vi "TDMS Channel Page.vi"(8 "error in (no error)":errorcluster, 11 "Node Ptr":T2 format="%.0x") -> (0 "error out":errorcluster)   [LabVIEW 2011, in "TDMS Custom Device.lvlib"]
uses:
  TDMS Custom Device.lvlib
  <vilib>/NI Veristand/Custom Device API/Custom Device Item Ref.ctl
  <vilib>/NI Veristand/Custom Device API/Get Item Property (Double).vi
  <vilib>/NI Veristand/Custom Device API/Get Item Property (I32).vi
  <vilib>/NI Veristand/Custom Device API/Get Item Property (Variant).vi
  <vilib>/NI Veristand/Custom Device API/Set Item Property (Double).vi
  <vilib>/NI Veristand/Custom Device API/Set Item Property (I32).vi
  <vilib>/NI Veristand/Custom Device API/Set Item Property (Variant).vi
  <vilib>/NI Veristand/Custom Device API/Custom Device API.lvlib
panel:
  in  "dt (sec)":dbl
  in  "Interpolation Width":i32=1 caption="The system uses this number of samples on either side of a point to be used by the above method. Increase to increase smoothness, decrease for performance." min=1 max=50
  in  "Interpolation Method":T1(ring)=enum."Linear"
  in  "Header":cluster{"Section Name":string}={"Section Name"="TDMS Channel Settings"}
  in  "Description":string
  out "Name":string
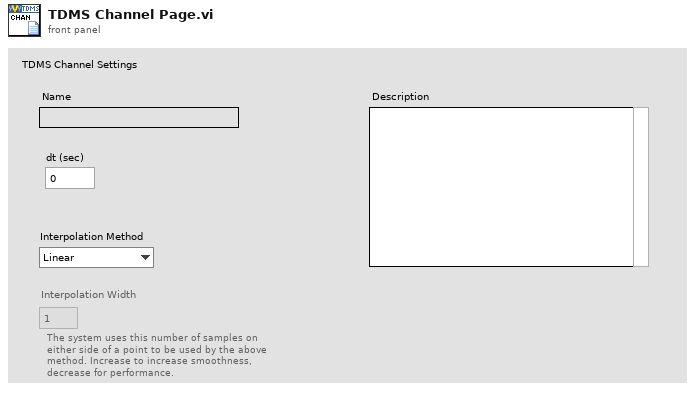
[diagram p1: front panel]
types:
  T1 = enum16{"Nearest", "Linear", "Spline", "Cubic Hermite", "Lagrange", "Polynomial"}
  T2 = typedef "Custom Device API.lvlib/Custom Device Item Ref.ctl" = u64
  T3 = enum8{"Enabled", "Disabled", "Disabled and Grayed Out"}
  T4 = typedef "Custom Device API.lvlib/Custom Device Item Info.ctl" = cluster{"Name":string, "Is Channel":bool, "GUID":string}
  T5 = typedef "Custom Device API.lvlib/Custom Device Commands.ctl" = enum16{"Default", "Item renamed", "Shutdown", "Dynamic button pressed"}
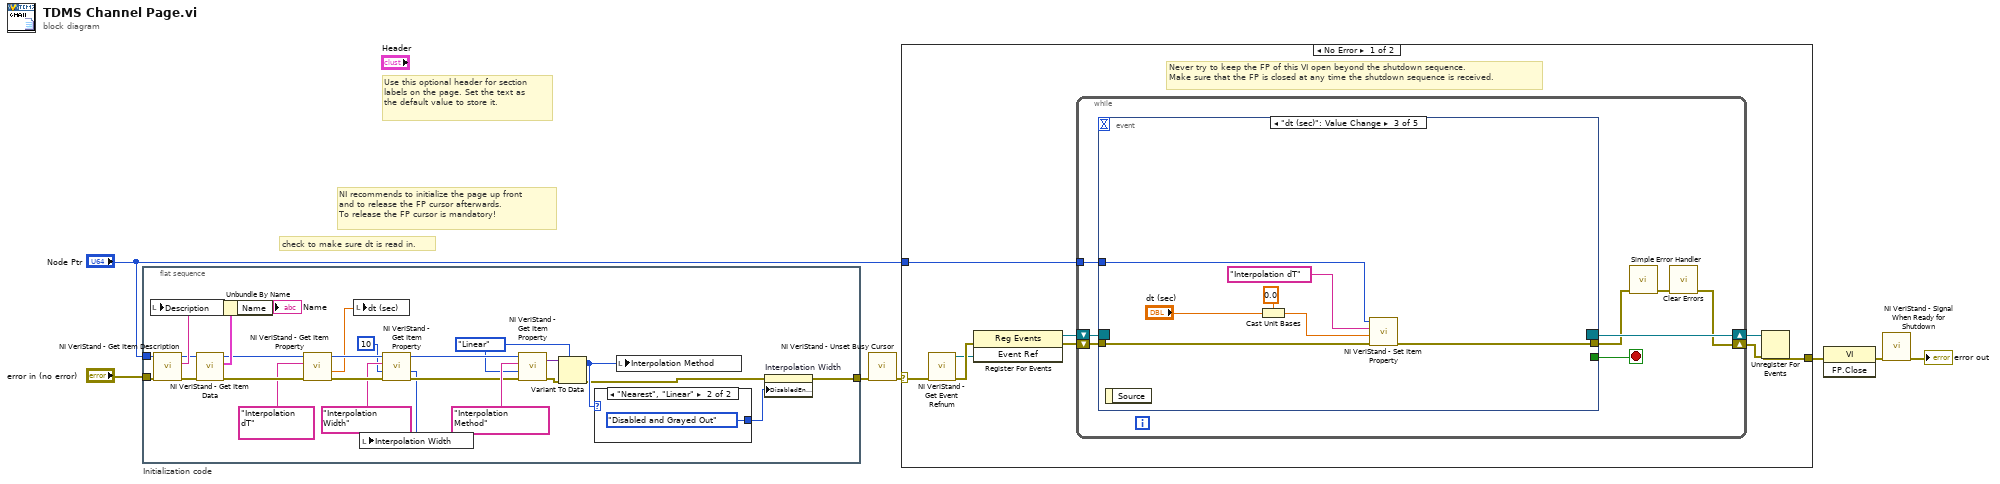
[diagram p0: block diagram]
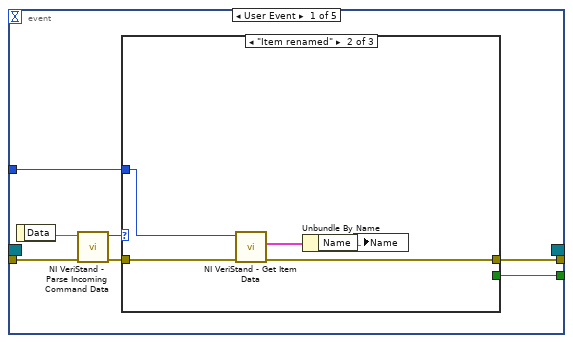
[diagram p2: hidden frame]
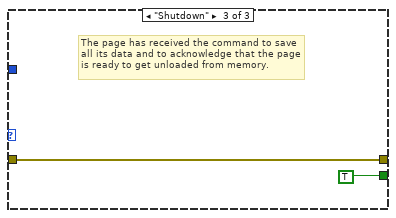
[diagram p4: hidden frame]
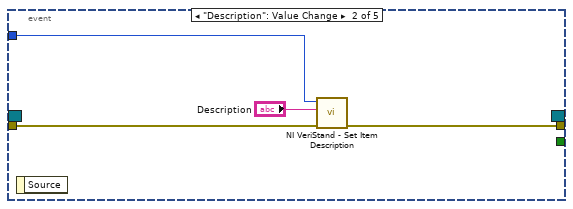
[diagram p5: hidden frame]
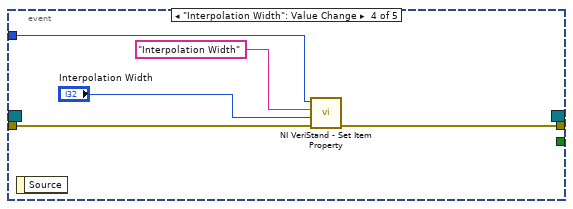
[diagram p6: hidden frame]
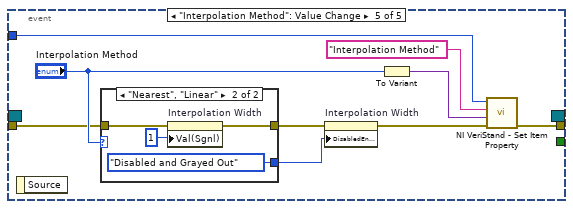
[diagram p7: hidden frame]
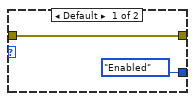
[diagram p8: hidden frame]
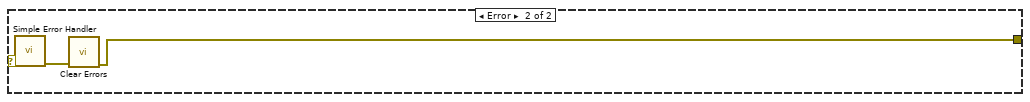
[diagram p9: hidden frame]
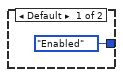
[diagram p10: hidden frame]
diagram:
  # "check to make sure dt is read in."
  # "Use this optional header for section labels on the page. Set the text as the default value to store it."
  # "NI recommends to initialize the page up front\nand to release the FP cursor afterwards.\nTo release the FP cursor is mandatory!"
  n1 = flat-sequence "Initialization code" {
    tunnel: "error in (no error)" -> [w33]
    tunnel: "Node Ptr" -> [w32]
    tunnel: [w12] -> w1
    frame #0 {
      w14 = T1."Linear" ("Interpolation Method")
      n2 = call <vilib>:"NI VeriStand - Get Item Description.vi"("error in (no error)"=w33, "Item Ref in"=w32) -> ("error out"=w30:errorcluster, "Description"=w31:string, "Item Ref out"=w29:T2)  [unwired: 7 out]
      n3 = local write "Description"(w31) -> ()
      n4 = call <vilib>:"NI VeriStand - Get Item Data.vi"("error in (no error)"=w30, "Item Ref in"=w29) -> ("error out"=w26:errorcluster, "Item Info"=w28:T4, "Item Ref out"=w27:T2)  [unwired: 7 out]
      n5 = Unbundle By Name(w28) -> ("Name"=→"Name":string)
      n6 = call-poly <vilib>:"NI VeriStand - Get Item Property.vi"("error in (no error)"=w26, "Property Name"="Interpolation dT", "Item Ref in"=w27) -> ("error out"=w20:errorcluster, "Value"=w8:dbl, "Item Ref out"=w19:T2)  [unwired: 1 in, 5 out]
      n7 = local write "dt (sec)"(w8) -> ()
      n8 = call-poly <vilib>:"NI VeriStand - Get Item Property.vi"("error in (no error)"=w20, "Default Value"=10, "Property Name"="Interpolation Width", "Item Ref in"=w19) -> ("error out"=w17:errorcluster, "Value"=w11:i32, "Item Ref out"=w18:T2)  [unwired: 5 out]
      n9 = local write "Interpolation Width"(w11) -> ()
      n10 = call-poly <vilib>:"NI VeriStand - Get Item Property.vi"("error in (no error)"=w17, "Default Value"=w14, "Property Name"="Interpolation Method", "Item Ref in"=w18) -> ("error out"=w21:errorcluster, "Value"=w22:variant)  [unwired: 6 out]
      n11 = Variant To Data(error in=w21, type=w14, Variant=w22) -> (data=w13:T1, error out=w10:errorcluster)
      n12 = case shown="\"Nearest\", \"Linear\"" w13 {
        tunnel: [T3."Enabled" ("Disabled") T3."Disabled and Grayed Out" ("Disabled")] -> w9
        frame Default {
        }
        frame "Nearest", "Linear" {
        }
      }
      n13 = local write "Interpolation Method"(w13) -> ()
      n14 = property on="Interpolation Width" class="DigNum (strict)"(error in=w10, "DisabledEnum"=w9) -> (error out=w12:errorcluster)  [unwired: 1 in, 1 out]
    }
  }
  n15 = call <vilib>:"NI VeriStand - Unset Busy Cursor.vi"("error in (no error)"=w1) -> ("error out"=w3:errorcluster)  [unwired: 10 out]
  n16 = case shown="No Error" w3 {
    selector: w3 -> [w36 w101]
    tunnel: [w41 w99] -> w7
    tunnel: "Node Ptr" -> [w37 _]
    frame No Error {
      # "Never try to keep the FP of this VI open beyond the shutdown sequence.\nMake sure that the FP is closed at any time the shutdown sequence is received."
      n17 = call <vilib>:"NI VeriStand - Get Event Refnum.vi"("error in (no error)"=w36) -> ("error out"=w44:errorcluster, "Event Ref"=w40:refnum<user-event>)  [unwired: 9 out]
      n18 = register-events(error in=w44, w40) -> (reference out=w38:refnum<event-registration>, error out=w39:errorcluster)  [unwired: 1 in]
      n19 = while {
        tunnel: w37 -> [w48]
        shift-right: [w45] -> w42
        shift-left: w39 -> [w51]
        shift-right: [w52] -> w43
        shift-left: w38 -> [w50]
        stop <- w49 stop-if-true
        n20 = event shown="[2] \"dt (sec)\": Value Change" {
          selector: w50 -> [_ _ _ _ _]
          dyn-events: [_ _ _ _ _] -> w52
          timeout: _ -> [_ _ _ _ _]
          tunnel: w51 -> [w59 w70 w78 w83 w87]
          tunnel: [w55 _ _ _ _] -> w49
          tunnel: [w54 w69 w77 w82 w88] -> w47
          tunnel: w48 -> [w53 w71 w76 w81 w92]
          event User Event {
            n21 = event-data() -> ("Data"=w58:string)  [unwired: 1 out]
            n22 = call <vilib>:"NI VeriStand - Parse Incoming Command Data.vi"("error in (no error)"=w59, "Incoming data"=w58) -> ("error out"=w57:errorcluster, "Action"=w56:T5)  [unwired: 8 out]
            n23 = case shown="\"Item renamed\"" w56 {
              tunnel: w57 -> [w60 w65 w66]
              tunnel: [_ _ TRUE] -> w55
              tunnel: [w60 w62 w66] -> w54
              tunnel: w53 -> [_ w64 _]
              frame "Default", Default {
              }
              frame "Item renamed" {
                n24 = call <vilib>:"NI VeriStand - Get Item Data.vi"("error in (no error)"=w65, "Item Ref in"=w64) -> ("error out"=w62:errorcluster, "Item Info"=w63:T4)  [unwired: 8 out]
                n25 = Unbundle By Name(w63) -> ("Name"=w61:string)
                n26 = local write "Name"(w61) -> ()
              }
              frame "Shutdown" {
                # "The page has received the command to save all its data and to acknowledge that the page is ready to get unloaded from memory."
              }
            }
          }
          event "Description": Value Change {
            n27 = event-data() -> ()  [unwired: 2 out]
            n28 = call <vilib>:"NI VeriStand - Set Item Description.vi"("error in (no error)"=w70, "Description"="Description", "Item Ref in"=w71) -> ("error out"=w69:errorcluster)  [unwired: 8 out]
          }
          event "dt (sec)": Value Change {
            n29 = event-data() -> ()  [unwired: 2 out]
            n30 = Cast Unit Bases(0:"dt (sec)", 1:0.0) -> (2:w74:dbl)
            n31 = call-poly <vilib>:"NI VeriStand - Set Item Property.vi"("error in (no error)"=w78, "Value"=w74, "Property Name"="Interpolation dT", "Item Ref in"=w76) -> ("error out"=w77:errorcluster)  [unwired: 7 out]
          }
          event "Interpolation Width": Value Change {
            n32 = event-data() -> ()  [unwired: 2 out]
            n33 = call-poly <vilib>:"NI VeriStand - Set Item Property.vi"("error in (no error)"=w83, "Value"="Interpolation Width", "Property Name"="Interpolation Width", "Item Ref in"=w81) -> ("error out"=w82:errorcluster)  [unwired: 7 out]
          }
          event "Interpolation Method": Value Change {
            n34 = event-data() -> ()  [unwired: 2 out]
            n35 = case shown="\"Nearest\", \"Linear\"" "Interpolation Method" {
              tunnel: [T3."Enabled" ("Disabled") T3."Disabled and Grayed Out" ("Disabled")] -> w84
              tunnel: w87 -> [w93 w96]
              tunnel: [w93 w95] -> w86
              frame Default {
              }
              frame "Nearest", "Linear" {
                n36 = property on="Interpolation Width" class="DigNum (strict)"(error in=w96, "Val(Sgnl)"=1 ("Value (Signaling)")) -> (error out=w95:errorcluster)  [unwired: 1 in, 1 out]
              }
            }
            n37 = property on="Interpolation Width" class="DigNum (strict)"(error in=w86, "DisabledEnum"=w84) -> (error out=w85:errorcluster)  [unwired: 1 in, 1 out]
            n38 = To Variant(anything="Interpolation Method") -> (Variant=w90:variant)
            n39 = call-poly <vilib>:"NI VeriStand - Set Item Property.vi"("error in (no error)"=w85, "Value"=w90, "Property Name"="Interpolation Method", "Item Ref in"=w92) -> ("error out"=w88:errorcluster)  [unwired: 7 out]
          }
        }
        n40 = call <vilib>:"Simple Error Handler.vi"("error in (no error)"=w47) -> ("error out"=w46:errorcluster)  [unwired: 1 in, 7 out]
        n41 = call <vilib>:"Clear Errors.vi"("error in (no error)"=w46) -> ("error out"=w45:errorcluster)  [unwired: 6 out]
      }
      n42 = Unregister For Events(event registration refnum=w43, error in=w42) -> (error out=w41:errorcluster)
    }
    frame Error {
      n43 = call <vilib>:"Simple Error Handler.vi"("error in (no error)"=w101) -> ("error out"=w100:errorcluster)  [unwired: 1 in, 7 out]
      n44 = call <vilib>:"Clear Errors.vi"("error in (no error)"=w100) -> ("error out"=w99:errorcluster)  [unwired: 6 out]
    }
  }
  n45 = invoke class="VI" method="FP.Close"(error in=w7) -> (error out=w6:errorcluster)  [unwired: 2 in, 2 out]
  n46 = call <vilib>:"NI VeriStand - Signal When Ready for Shutdown.vi"("error in (no error)"=w6) -> ("error out"=→"error out":errorcluster)  [unwired: 10 out]
